vi "emi_int Changed w init.vi"(7 "x":i32, 13 "Initial(0)":i32) -> (6 "Rising":bool, 8 "changed":bool, 10 "Falling":bool)   [LabVIEW 2010]
doc: "Monitors a int 32, indicateing change, and wheter it was rising or falling. \n\nOn first call, it reads the Initial input, and uses that as the previous value for comparison.\n\nreentrant Subroutine."
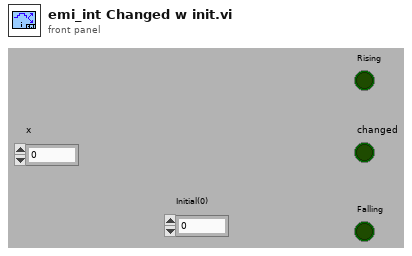
[diagram p1: front panel]
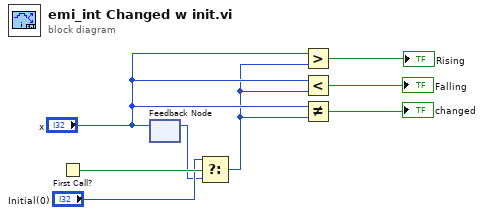
[diagram p0: block diagram]
diagram:
  n1 = First Call?() -> (First Call?: T/F=w8:bool)
  n2 = feedback-in #1("x") -> ()
  n3 = feedback #1() -> (w5:i32)  [unwired: 1 in]
  n4 = Select(t="Initial(0)", s=w8, f=w5) -> (s? t:f=w3:i32)
  n5 = Greater?(x="x", y=w3) -> (0:→"Rising":bool)
  n6 = Less?(x="x", y=w3) -> (x < y?=→"Falling":bool)
  n7 = Not Equal?(x="x", y=w3) -> (x != y?=→"changed":bool)
